vi "Message to Display String.vi"(1 "Message":T1) -> (0 "message string":string)   [LabVIEW 2019, in "RemoteControl.lvlib" / "RemoteControl.lvclass"]
uses:
  RemoteControl.lvclass
  Typedefs/Message--Cluster.ctl
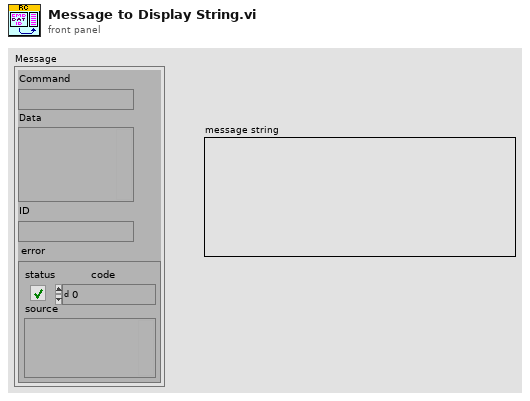
[diagram p1: front panel]
types:
  T1 = typedef "RemoteControl.lvlib/RemoteControl.lvclass/Message--Cluster.ctl" = cluster{"Command":string, "Data":variant, "ID":string, "error":errorcluster}
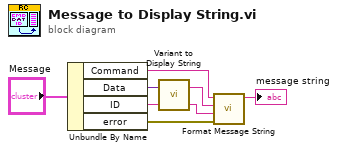
[diagram p0: block diagram]
diagram:
  n1 = Unbundle By Name("Message") -> ("Command"=w5:string, "Data"=w6:variant, "ID"=w3:string, "error"=w1:errorcluster)
  n2 = call "Variant to Display String.vi"("Variant"=w6) -> ("xml string"=w2:string)  [unwired: 2 in]
  n3 = call "Format Message String.vi"("error"=w1, "ID"=w3, "Data"=w2, "Command"=w5) -> ("Message"=→"message string":string)  [unwired: 7 in]
